vi "Write Attributes.vi"(4 "Actor Ref":refnum<vi>, 5 "Alias":string, 6 "Creator Attributes":refnum<class "Attributes.lvclass">, 7 "Unified Msg Set":T1, 9 "Queue of Self Attributes":refnum<queue>, 10 "Queue of Error":refnum<queue>, 11 "Base Actor in":refnum<class "Base Actor.lvclass">) -> (0 "Error out":errorcluster, 3 "Base Actor out":refnum<class "Base Actor.lvclass">)   [LabVIEW 2020, in "jettl.lvlib" / "Actor.lvlib" / "Base Actor.lvclass"]
uses:
  Base Actor.lvclass
  Attributes/Attributes/Attributes.lvclass
  Msg Set.ctl
  Msg/Msg.lvclass
  Base Actor.lvclass/Base Actor.ctl
  Attributes/Attributes.lvlib
  Actor.lvlib
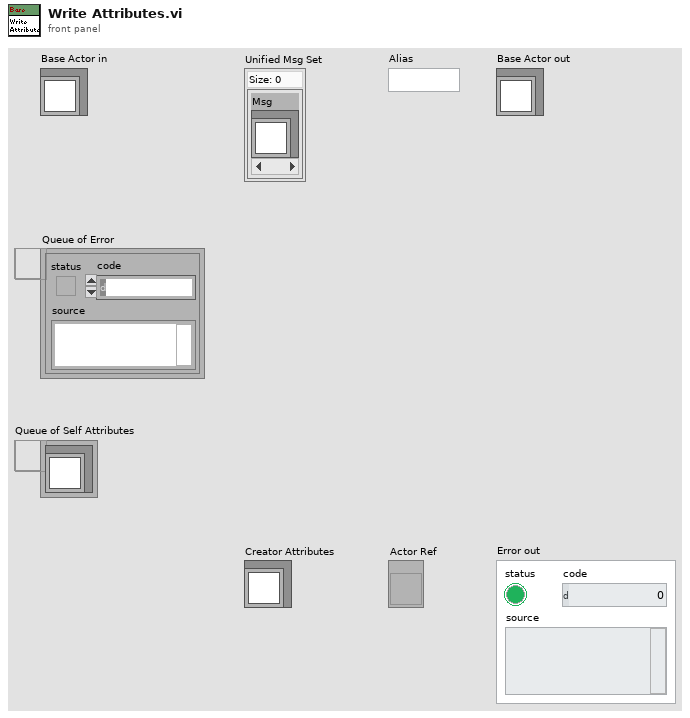
[diagram p1: front panel]
types:
  T1 = typedef "jettl.lvlib/Actor.lvlib/Msg Set.ctl" = set{refnum<class "Msg.lvclass">}
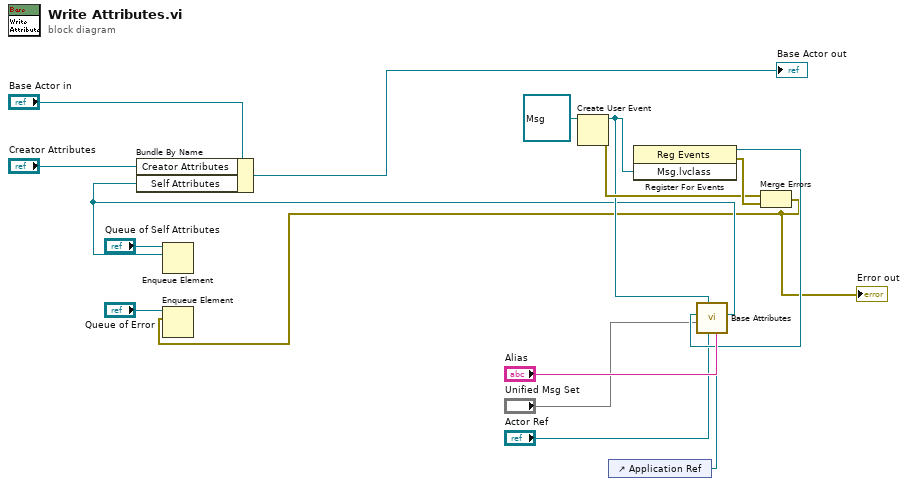
[diagram p0: block diagram]
diagram:
  n1 = Create User Event(user event datatype=refnum<class "Msg.lvclass"> refnum ("Msg.lvclass")) -> (user event=w8:refnum<user-event>, error out=w11:errorcluster)  [unwired: 1 in]
  n2 = control-ref of="Application Ref"() -> (w6:refnum<vi>)
  n3 = register-events(w8) -> (reference out=w7:refnum<event-registration>, error out=w12:errorcluster)  [unwired: 2 in]
  n4 = call "Base Attributes.vi"("Application Ref"=w6, "Alias"="Alias", "Actor Ref"="Actor Ref", "Address"=w8, "Unified Msg Set"="Unified Msg Set", "Event Ref"=w7) -> ("Attributes"=w4:refnum<class "Attributes.lvclass">)  [unwired: 5 in]
  n5 = Bundle By Name(cluster="Base Actor in", "Creator Attributes"="Creator Attributes", "Self Attributes"=w4) -> (→"Base Actor out":refnum<class "Base Actor.lvclass">)
  n6 = Enqueue Element(queue="Queue of Self Attributes", element=w4) -> ()  [unwired: 2 in, 3 out]
  n7 = Merge Errors(w11, w12) -> (w1:errorcluster)
  "Error out" <- w1
  n8 = Enqueue Element(queue="Queue of Error", element=w1) -> ()  [unwired: 2 in, 3 out]
